vi "Calculate Movement Duration for Linear Motion Profile.vi"(0 "Cluster in":T5, 11 "error in":errorcluster) -> (4 "Cluster out":T5, 15 "error out":errorcluster)   [LabVIEW 2019, in "Motion Profile Generator.lvclass"]
uses:
  Motion Profile Generator.lvclass
  Type Defs/Ramp - Final Snapshot Request.ctl
  Type Defs/Ramp - Velocity and Acceleration Mode.ctl
  Type Defs/Motion Snapshot.ctl
  Type Defs/Control Boundaries.ctl
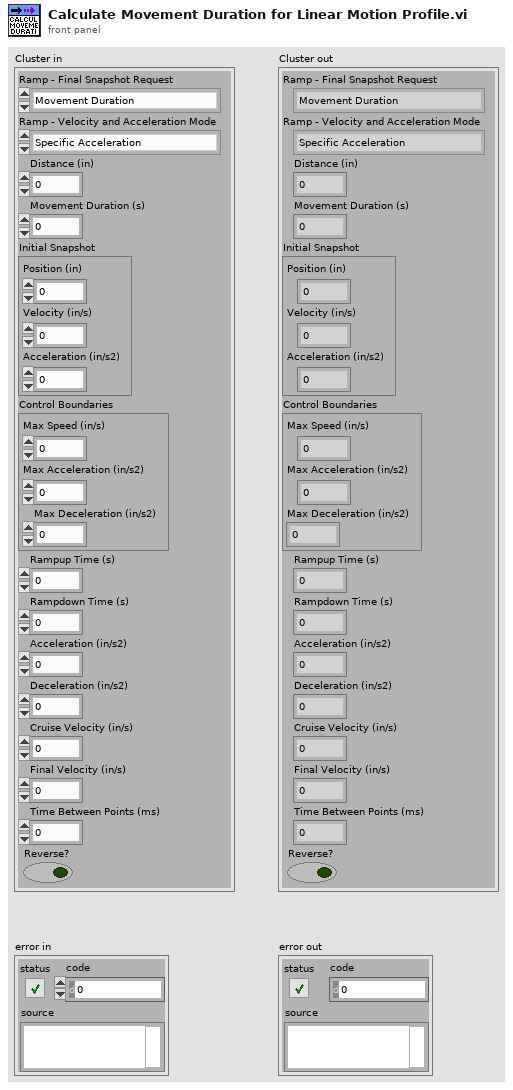
[diagram p1: front panel]
types:
  T1 = typedef "Motion Profile Generator.lvclass/Ramp - Final Snapshot Request.ctl" = enum16{"Movement Duration", "Distance"}
  T2 = typedef "Motion Profile Generator.lvclass/Ramp - Velocity and Acceleration Mode.ctl" = enum16{"Specific Acceleration", "Rampup and Rampdown Times"}
  T3 = typedef "Motion Profile Generator.lvclass/Motion Snapshot.ctl" = cluster{"Position (in)":dbl, "Velocity (in/s)":dbl, "Acceleration (in/s2)":dbl}
  T4 = typedef "Motion Profile Generator.lvclass/Control Boundaries.ctl" = cluster{"Max Speed (in/s)":dbl, "Max Acceleration (in/s2)":dbl, "Max Deceleration (in/s2)":dbl}
  T5 = cluster{"Ramp - Final Snapshot Request":T1, "Ramp - Velocity and Acceleration Mode":T2, "Distance (in)":dbl, "Movement Duration (s)":dbl, "Initial Snapshot":T3, "Control Boundaries":T4, "Rampup Time (s)":dbl, "Rampdown Time (s)":dbl, "Acceleration (in/s2)":dbl, "Deceleration (in/s2)":dbl, "Cruise Velocity (in/s)":dbl, "Final Velocity (in/s)":dbl, "Time Between Points (ms)":dbl, "Reverse?":bool}
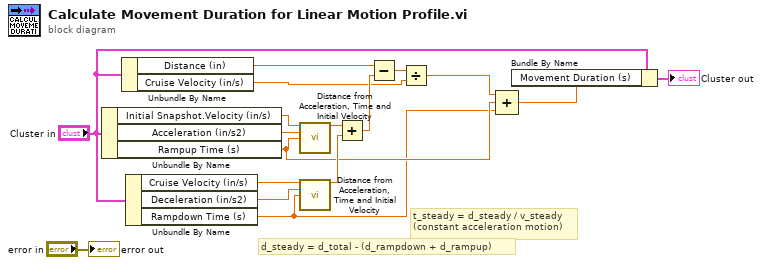
[diagram p0: block diagram]
diagram:
  # "d_steady = d_total - (d_rampdown + d_rampup)"
  # "t_steady = d_steady / v_steady\n(constant acceleration motion)"
  n1 = Unbundle By Name("Cluster in") -> ("Initial Snapshot.Velocity (in/s)"=w15:dbl, "Acceleration (in/s2)"=w14:dbl, "Rampup Time (s)"=w3:dbl)
  n2 = Unbundle By Name("Cluster in") -> ("Distance (in)"=w8:dbl, "Cruise Velocity (in/s)"=w5:dbl)
  n3 = Unbundle By Name("Cluster in") -> ("Cruise Velocity (in/s)"=w12:dbl, "Deceleration (in/s2)"=w13:dbl, "Rampdown Time (s)"=w2:dbl)
  n4 = call "Distance from Acceleration, Time and Initial Velocity.vi"("Initial Velocity (in/s)"=w15, "Acceleration (in/s2)"=w14, "Time (s)"=w3) -> ("Distance (in)"=w10:dbl)  [unwired: 11 in, 1 out]
  n5 = call "Distance from Acceleration, Time and Initial Velocity.vi"("Initial Velocity (in/s)"=w12, "Acceleration (in/s2)"=w13, "Time (s)"=w2) -> ("Distance (in)"=w9:dbl)  [unwired: 11 in, 1 out]
  n6 = Add(x=w10, y=w9) -> (x+y=w7:dbl)
  n7 = Subtract(x=w8, y=w7) -> (x-y=w6:dbl)
  n8 = Divide(x=w6, y=w5) -> (x/y=w4:dbl)
  n9 = Compound Arithmetic op=ADD(w4, w3, w2) -> (w1:dbl)
  n10 = Bundle By Name(cluster="Cluster in", "Movement Duration (s)"=w1) -> (→"Cluster out":T5)
  "error out" <- "error in"
